vi "White Noise.vi"(5 "Amplitude (V)":dbl=1.0 max=19.0 step=1.0, 6 "Stimulation freq (stim/sec)":u32=20, 7 "Fs (#S/s)":dbl=200000.0) -> (0 "Stimulus Waveform":waveform(dbl)(graph), 1 "Stimulus duration (ms)":dbl, 2 "Delay (ms)":dbl=1.0, 3 "Signal duration (#S)":dbl, 4 "Signal duration (ms)":dbl)   [LabVIEW 2014]
uses:
  <vilib>/Analysis/1siggen.llb/Ramp Pattern by Samples.vi
  <vilib>/Analysis/NI_AALBase.lvlib
panel:
  out "Amplitude (1/10 V)":dbl
  out "Plateu duration (#S)":dbl
  out "Ramp duration (#S)":dbl
  in  "start":dbl
  out "end":dbl
  out "Delay (#S)":dbl
  in  "Plateu duration (ms)":dbl=10.0
  in  "Ramp duration (ms)":dbl=1.0
  # "Stimulus Configuration"
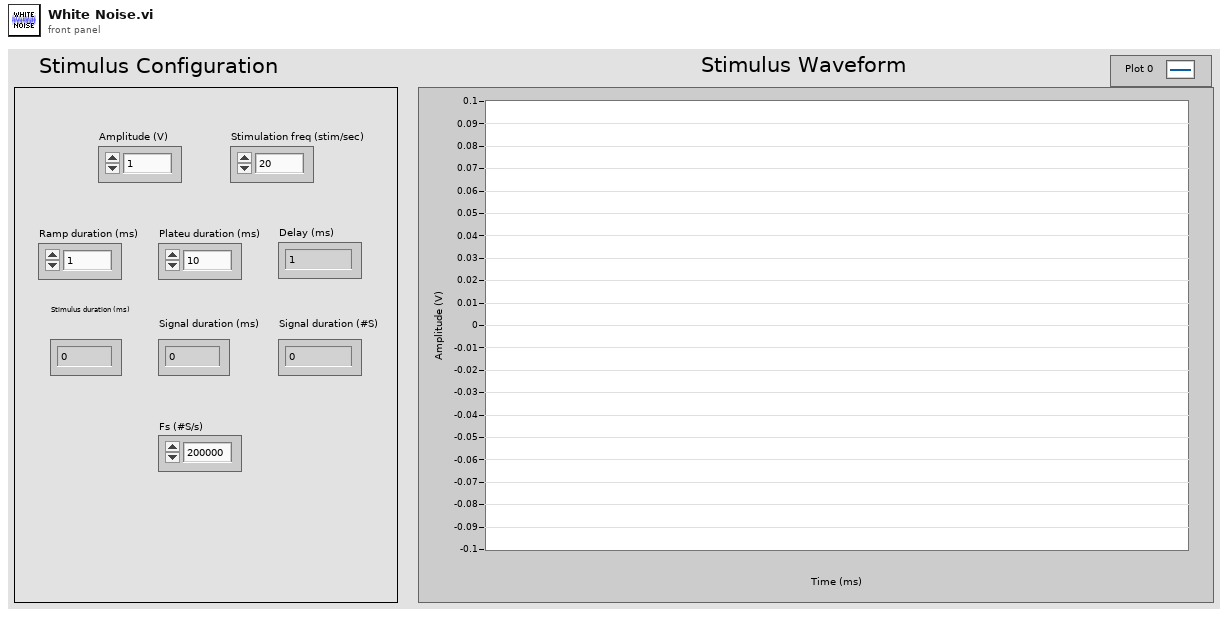
[diagram p1: front panel]
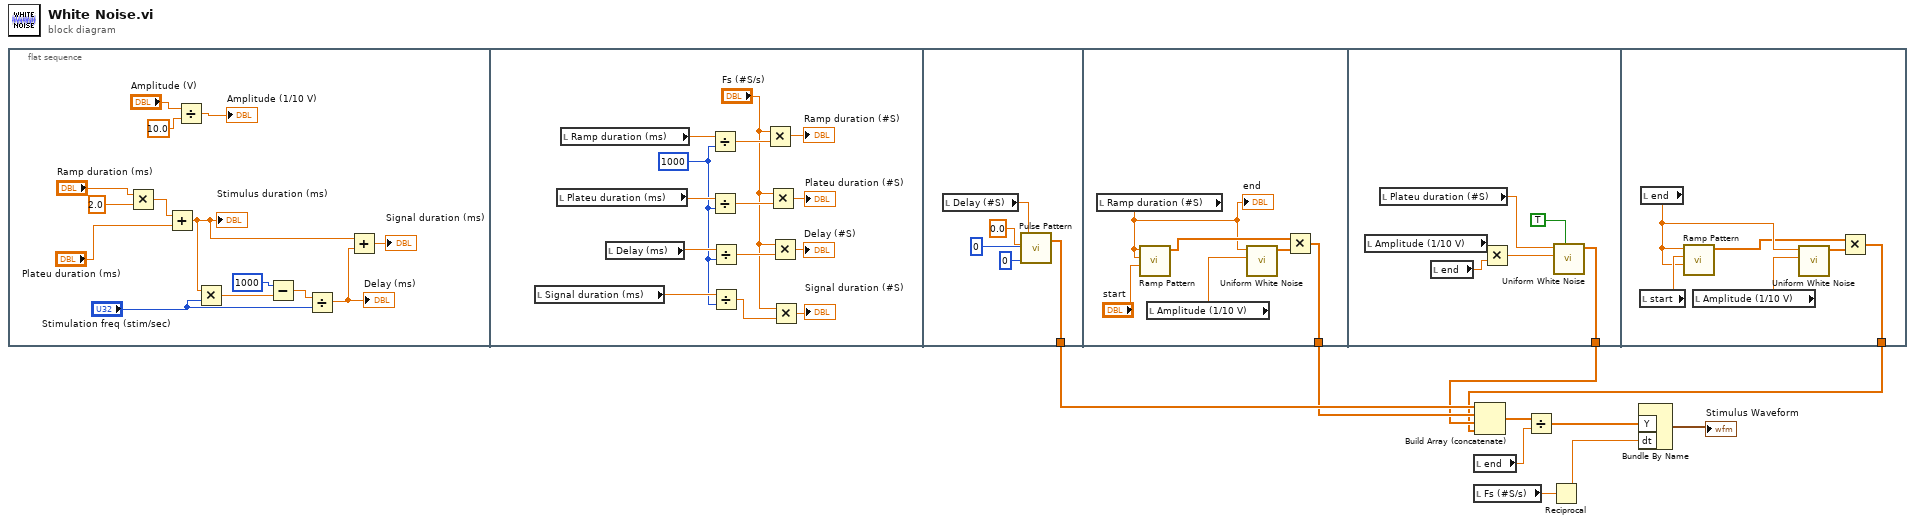
[diagram p0: block diagram]
diagram:
  n1 = flat-sequence {
    tunnel: [w39] -> w9
    tunnel: [w45] -> w8
    tunnel: [w50] -> w7
    tunnel: [w56] -> w6
    frame #0 {
      n2 = Multiply(x="Ramp duration (ms)", y=2.0) -> (x*y=w19:dbl)
      n3 = Add(x=w19, y="Plateu duration (ms)") -> (x+y=w12:dbl)
      "Stimulus duration (ms)" <- w12
      n4 = Divide(x="Amplitude (V)", y=10.0) -> (x/y=→"Amplitude (1/10 V)":dbl)
      n5 = Multiply(x=w12, y="Stimulation freq (stim/sec)") -> (x*y=w15:dbl)
      n6 = Subtract(x=1000, y=w15) -> (x-y=w16:dbl)
      n7 = Divide(x=w16, y="Stimulation freq (stim/sec)") -> (x/y=w11:dbl)
      "Delay (ms)" <- w11
      n8 = Add(x=w12, y=w11) -> (x+y=→"Signal duration (ms)":dbl)
    }
    frame #1 {
      w28 = 1000
      n9 = local read "Signal duration (ms)"() -> (w29:dbl)
      n10 = local read "Plateu duration (ms)"() -> (w35:dbl)
      n11 = local read "Ramp duration (ms)"() -> (w38:dbl)
      n12 = local read "Delay (ms)"() -> (w34:dbl)
      n13 = Divide(x=w38, y=w28) -> (x/y=w36:dbl)
      n14 = Divide(x=w35, y=w28) -> (x/y=w32:dbl)
      n15 = Divide(x=w34, y=w28) -> (x/y=w30:dbl)
      n16 = Divide(x=w29, y=w28) -> (x/y=w25:dbl)
      n17 = Multiply(x="Fs (#S/s)", y=w36) -> (x*y=→"Ramp duration (#S)":dbl)
      n18 = Multiply(x="Fs (#S/s)", y=w32) -> (x*y=→"Plateu duration (#S)":dbl)
      n19 = Multiply(x="Fs (#S/s)", y=w30) -> (x*y=→"Delay (#S)":dbl)
      n20 = Multiply(x="Fs (#S/s)", y=w25) -> (x*y=→"Signal duration (#S)":dbl)
    }
    frame #2 {
      n21 = local read "Delay (#S)"() -> (w43:dbl)
      n22 = call <vilib>:"Pulse Pattern.vi"("width"=0, "delay"=0, "amplitude"=0.0, "samples"=w43) -> ("Pulse Pattern"=w39:dbl[])  [unwired: 1 out]
    }
    frame #3 {
      n23 = local read "Ramp duration (#S)"() -> (w44:dbl)
      "end" <- w44
      n24 = call-poly <vilib>:"Ramp Pattern.vi"("start"="start", "end"=w44, "samples"=w44) -> ("Ramp Pattern"=w46:dbl[])  [unwired: 7 in, 1 out]
      n25 = local read "Amplitude (1/10 V)"() -> (w48:dbl)
      n26 = call <vilib>:"Uniform White Noise.vi"("amplitude"=w48, "samples"=w44) -> ("uniform white noise"=w47:dbl[])  [unwired: 8 in, 1 out]
      n27 = Multiply(x=w46, y=w47) -> (x*y=w45:dbl[])
    }
    frame #4 {
      n28 = local read "Amplitude (1/10 V)"() -> (w54:dbl)
      n29 = local read "Plateu duration (#S)"() -> (w55:dbl)
      n30 = local read "end"() -> (w53:dbl)
      n31 = Multiply(x=w54, y=w53) -> (x*y=w52:dbl)
      n32 = call <vilib>:"Uniform White Noise.vi"("initialize?"=TRUE ("reset phase"), "amplitude"=w52, "samples"=w55) -> ("uniform white noise"=w50:dbl[])  [unwired: 7 in, 1 out]
    }
    frame #5 {
      n33 = local read "start"() -> (w61:dbl)
      n34 = local read "end"() -> (w60:dbl)
      n35 = call-poly <vilib>:"Ramp Pattern.vi"("start"=w60, "end"=w61, "samples"=w60) -> ("Ramp Pattern"=w57:dbl[])  [unwired: 7 in, 1 out]
      n36 = local read "Amplitude (1/10 V)"() -> (w59:dbl)
      n37 = call <vilib>:"Uniform White Noise.vi"("amplitude"=w59, "samples"=w60) -> ("uniform white noise"=w58:dbl[])  [unwired: 8 in, 1 out]
      n38 = Multiply(x=w57, y=w58) -> (x*y=w56:dbl[])
    }
  }
  n39 = local read "end"() -> (w4:dbl)
  n40 = local read "Fs (#S/s)"() -> (w2:dbl)
  n41 = Build Array (concatenate)(w9, w8, w7, w6) -> (w5:dbl[])
  n42 = Divide(x=w5, y=w4) -> (x/y=w3:dbl[])
  n43 = Reciprocal(x=w2) -> (1/x=w1:dbl)
  n44 = Bundle By Name("Y"=w3, "dt"=w1) -> (→"Stimulus Waveform":waveform(dbl))  [unwired: 1 in]
